vi "KE3706A_Test.vi"(8 "error in (no error)":errorcluster, 11 "KE3706A in":refnum<class "KE3706A.lvclass">) -> (0 "error out":errorcluster, 3 "KE3706A out":refnum<class "KE3706A.lvclass">)   [LabVIEW 2013, in "KE3706A.lvclass"]
uses:
  KE3706A.lvclass
  <vilib>/Platform/TimedLoop/XDataNode/timing_clust.ctl
  <vilib>/Platform/TimedLoop/XDataNode/nitl_modes.ctl
  <vilib>/Platform/TimedLoop/XDataNode/wakeup.ctl
  InstrumentSetup.vi
  <vilib>/platform/TimedLoop/XDataNode/XDataNode.xnode
  <vilib>/Platform/TimedLoop/XDataNode/XDNodeRunTimeDep.lvlib
  InstrControl.lvclass
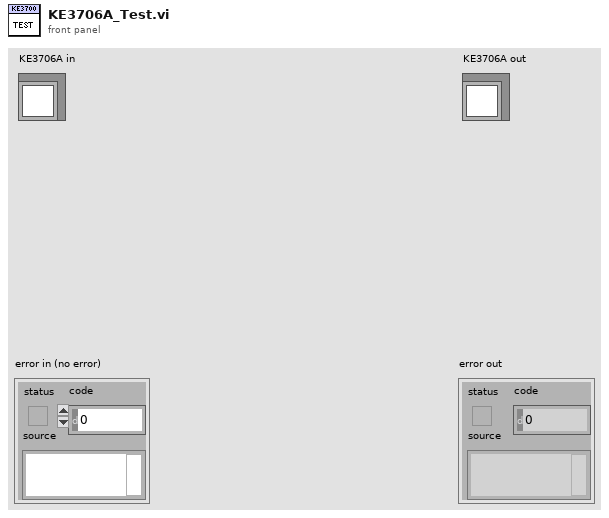
[diagram p1: front panel]
types:
  T1 = cluster{"KE 2410":cluster{"Instrument name":string, "address":refnum<visa-resource-name>, "Instrument type":u16}, "KE 2410_2":cluster{"Instrument name":string, "address":refnum<visa-resource-name>, "Instrument type":u16}, "KE 6517":cluster{"Instrument name":string, "address":refnum<visa-resource-name>, "Instrument type":u16}, "KE 6517_2":cluster{"Instrument name":string, "address":refnum<visa-resource-name>, "Instrument type":u16}, "KE 487":cluster{"Instrument name":string, "address":refnum<visa-resource-name>, "Instrument type":u16}, "KE 236":cluster{"Instrument name":string, "address":refnum<visa-resource-name>, "Instrument type":u16}, "WK 6440B":cluster{"Instrument name":string, "address":refnum<visa-resource-name>, "Instrument type":u16}, "WK 6425":cluster{"Instrument name":string, "address":refnum<visa-resource-name>, "Instrument type":u16}, "HP 4263B":cluster{"Instrument name":string, "address":refnum<visa-resource-name>, "Instrument type":u16}, "Pickering Matrix":cluster{"Instrument name":string, "address":refnum<visa-resource-name>, "Instrument type":u16}, "KE 2000":cluster{"Instrument name":string, "address":refnum<visa-resource-name>, "Instrument type":u16}, "KE3706A Switching":cluster{"Instrument name":string, "address":refnum<visa-resource-name>, "Instrument type":u16}}
  T2 = cluster{"Mux1 slot":string, "Mux2 slot":string, "KE3706A":refnum<class "KE3706A.lvclass">}
  T3 = typedef "XDNodeRunTimeDep.lvlib/timing_clust.ctl" = cluster{"Expected End [f-1]":u64, "Actual End [f-1]":u64, "Finished Late? [f-1]":bool, "Expected End [i-1]":u64, "Actual End [i-1]":u64, "Finished Late? [i-1]":bool, "Expected Start [i]":u64, "Actual Start [i]":u64, "Expected Start [f]":u64, "Actual Start [f]":u64, "Source Name":string, "Structure Name":string, "Period":i64, "Deadline":i64, "Offset":i64, "Start":i64, "Priority":i32, "Timeout":i32, "Mode":T4, "Wakeup Reason":T5, "Error":errorcluster, "Source Type":string, "Secondary Source Type":string, "Global End Time":u64, "Global Start Time":u64, "Frame Duration":u64, "Iteration Duration":u64, "Assigned CPU":i32, "I/O Scan Engine Mode":u32}
  T4 = typedef "XDNodeRunTimeDep.lvlib/nitl_modes.ctl" = enum32{"No Change", "Process missed periods, maintain original phase", "Discard missed periods, maintain original phase", "Process missed periods, ignore original phase", "Discard missed periods, ignore original phase"}
  T5 = typedef "XDNodeRunTimeDep.lvlib/wakeup.ctl" = enum32{"Normal", "Aborted", "Asynchronous wakeup", "Timing source error", "Timed loop error", "Timeout"}
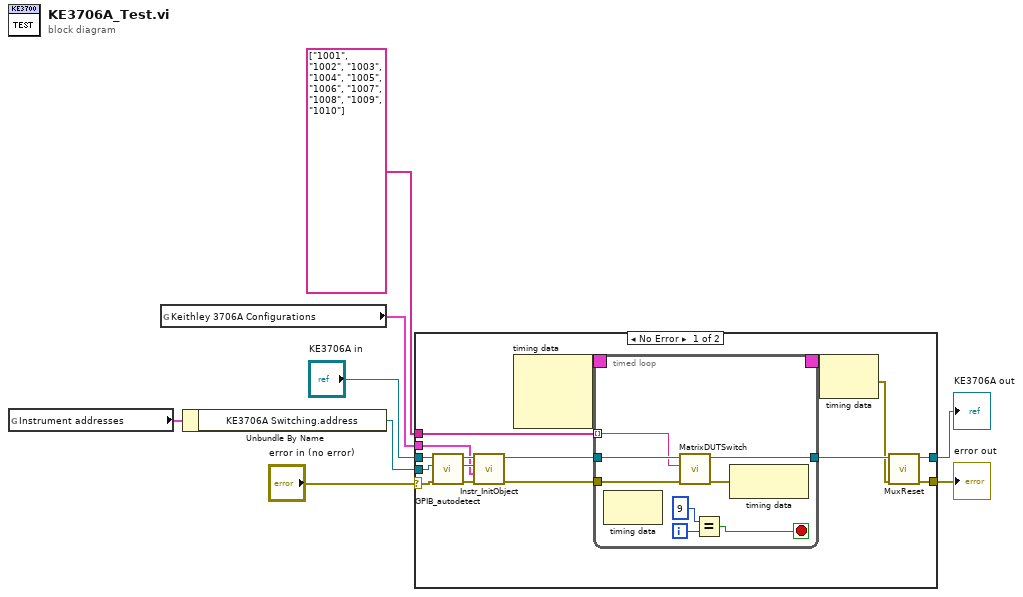
[diagram p0: block diagram]
diagram:
  n1 = global read "InstrumentSetup.vi" "Instrument addresses"() -> (w2:T1)
  n2 = global read "InstrumentSetup.vi" "Keithley 3706A Configurations"() -> (w3:T2)
  n3 = Unbundle By Name(w2) -> ("KE3706A Switching.address"=w1:refnum<visa-resource-name>)
  n4 = case shown="No Error" "error in (no error)" {
    selector: "error in (no error)" -> [w13 w41]
    tunnel: [w9 w41] -> w7
    tunnel: [w10 w40] -> w5
    tunnel: "KE3706A in" -> [w19 w40]
    tunnel: string[] ["1001", "1002", "1003", "1004", "1005", "1006", "1007", "1008", "1009", "1010"] -> [w18 _]
    tunnel: w3 -> [w15 _]
    tunnel: w1 -> [w12 _]
    frame No Error {
      n5 = call-dynamic "GPIB_autodetect.vi"("error in (no error)"=w13, "Instrument address in"=w12, "InstrControl in"=w19) -> ("error out"=w21:errorcluster, "Instrument address out"=w22:refnum<visa-resource-name>, "InstrControl out"=w20:refnum<class "KE3706A.lvclass">)  [unwired: 6 in]
      n6 = call-dynamic "Instr_InitObject.vi"("error in (no error)"=w21, "Instrument Configuration"=w15, "Instrument address"=w22, "KE3700A in"=w20) -> ("error out"=w17:errorcluster, "KE3700A out"=w16:refnum<class "KE3706A.lvclass">)  [unwired: 6 in]
      n7 = node-c288() -> (w24:T3)  [unwired: 3 in]
      n8 = timed-loop {
        timing: w24 -> [_]
        timing-out: [_] -> w23
        tunnel: w18 -> [w27] mode=indexing
        tunnel: w17 -> [w32]
        tunnel: w16 -> [w28]
        tunnel: [w26] -> w14
        i -> [w30]
        stop <- w29 stop-if-true
        n9 = node-c288() -> ()  [unwired: 1 in, 1 out]
        n10 = call-dynamic "MatrixDUTSwitch.vi"("error in (no error)"=w32, "Channel #"=w27, "KE3700A in"=w28) -> ("error out"=w25:errorcluster, "KE3700A out"=w26:refnum<class "KE3706A.lvclass">)  [unwired: 7 in]
        n11 = Equal?(x=9, y=w30) -> (x = y?=w29:bool)
        n12 = node-c288(w25) -> ()  [unwired: 1 out]
      }
      n13 = node-c288(w23) -> (w11:errorcluster)
      n14 = call-dynamic "MuxReset.vi"("error in (no error)"=w11, "KE3700A in"=w14) -> ("error out"=w9:errorcluster, "KE3700A out"=w10:refnum<class "KE3706A.lvclass">)  [unwired: 8 in]
    }
    frame Error {
    }
  }
  "error out" <- w7
  "KE3706A out" <- w5
